vi "stop-machine-global.vi"() -> ()   [LabVIEW 2013]
panel:
  in  "Stop machine":bool
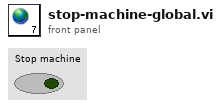
[diagram p1: front panel]
diagram:
